vi "Close All Control Refnums.vi"(8 "error in (no error)":errorcluster, 11 "Cluster":T1) -> (0 "error out":errorcluster)   [LabVIEW 2018]
uses:
  Control Refnum Cluster.ctl
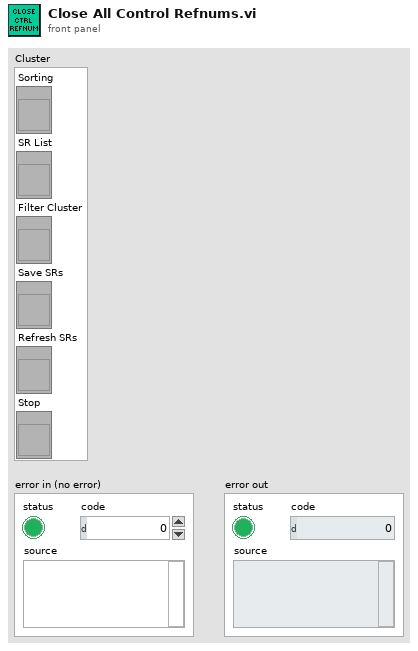
[diagram p1: front panel]
types:
  T1 = typedef "Control Refnum Cluster.ctl" = cluster{"Sorting":refnum<vi>, "SR List":refnum<vi>, "Filter Cluster":refnum<vi>, "Save SRs":refnum<vi>, "Refresh SRs":refnum<vi>, "Stop":refnum<vi>}
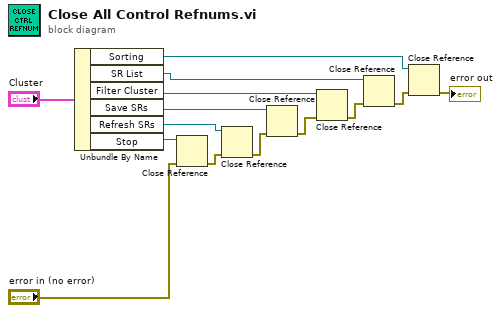
[diagram p0: block diagram]
diagram:
  n1 = Unbundle By Name("Cluster") -> ("Sorting"=w13:refnum<vi>, "SR List"=w12:refnum<vi>, "Filter Cluster"=w9:refnum<vi>, "Save SRs"=w8:refnum<vi>, "Refresh SRs"=w7:refnum<vi>, "Stop"=w6:refnum<vi>)
  n2 = Close Reference(reference=w6, error in (no error)="error in (no error)") -> (error out=w4:errorcluster)
  n3 = Close Reference(reference=w7, error in (no error)=w4) -> (error out=w3:errorcluster)
  n4 = Close Reference(reference=w8, error in (no error)=w3) -> (error out=w5:errorcluster)
  n5 = Close Reference(reference=w9, error in (no error)=w5) -> (error out=w10:errorcluster)
  n6 = Close Reference(reference=w12, error in (no error)=w10) -> (error out=w11:errorcluster)
  n7 = Close Reference(reference=w13, error in (no error)=w11) -> (error out=→"error out":errorcluster)
